vi "ListScript.vi"(10 "Params":variant, 11 "ScriptLine":string) -> ()   [LabVIEW 2014, in "Test.lvclass"]
uses:
  Test.lvclass
panel:
  out "List":string
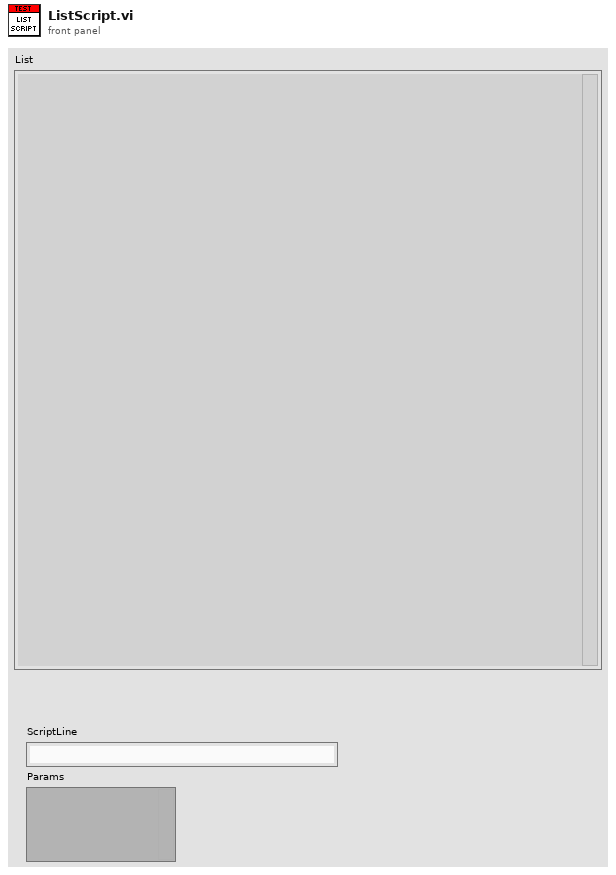
[diagram p1: front panel]
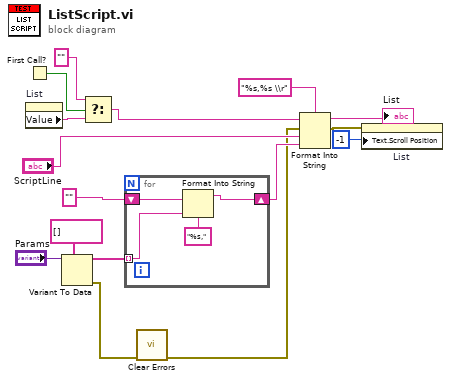
[diagram p0: block diagram]
diagram:
  n1 = First Call?() -> (First Call?: T/F=w12:bool)
  n2 = property on="List" class="Str"() -> ("Value"=w13:string)  [unwired: 2 in, 2 out]
  n3 = Variant To Data(type=string[] [], Variant="Params") -> (data=w7:string[], error out=w4:errorcluster)  [unwired: 1 in]
  n4 = Select(t="", s=w12, f=w13) -> (s? t:f=w10:string)
  n5 = for {
    tunnel: w7 -> [w18] mode=indexing
    shift-right: [w17] -> w5
    shift-left: "" -> [w19]
    n6 = Format Into String(format string="%s,", initial string=w19, w18) -> (resulting string=w17:string)  [unwired: 1 in, 1 out]
  }
  n7 = call <vilib>:"Clear Errors.vi"("error in (no error)"=w4) -> ("error out"=w3:errorcluster)  [unwired: 5 in, 1 out]
  n8 = Format Into String(format string="%s,%s \\r", initial string=w10, error in=w3, "ScriptLine", w5) -> (resulting string=→"List":string, error out=w1:errorcluster)
  n9 = property on="List" class="Str"(error in=w1, "Text.Scroll Position"=-1) -> ()  [unwired: 1 in, 2 out]
